vi "FlatToRichcif_manager_ClockUpdate.vi"(5 "OutputClusterType":T1, 11 "InputCluster":T3) -> (3 "OutputCluster":T1)   [LabVIEW 2021, in "CIF_Launcher_client.lvlib"]
uses:
  CIF_Launcher_client.lvlib
  cif_manager_ClockUpdate_Flat.ctl
  cif_manager_TimePair_Flat.ctl
  cif_manager_ClockUpdate.ctl
  cif_manager_TimePair.ctl
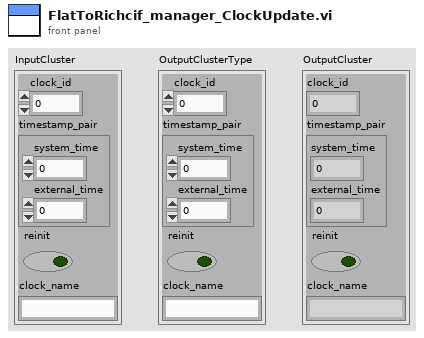
[diagram p1: front panel]
types:
  T1 = typedef "CIF_Launcher_client.lvlib/cif_manager_ClockUpdate.ctl" = cluster{"clock_id":u32, "timestamp_pair":T2, "reinit":bool, "clock_name":string}
  T2 = typedef "CIF_Launcher_client.lvlib/cif_manager_TimePair.ctl" = cluster{"system_time":i64, "external_time":i64}
  T3 = typedef "CIF_Launcher_client.lvlib/cif_manager_ClockUpdate_Flat.ctl" = cluster{"clock_id":u32, "timestamp_pair":T4, "reinit":bool, "clock_name":string}
  T4 = typedef "CIF_Launcher_client.lvlib/cif_manager_TimePair_Flat.ctl" = cluster{"system_time":i64, "external_time":i64}
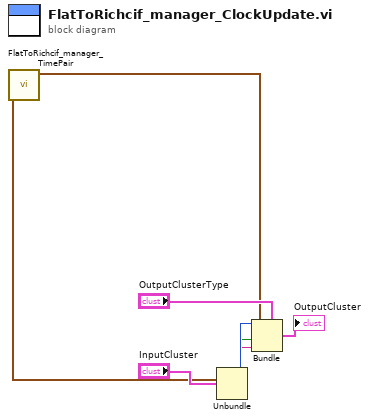
[diagram p0: block diagram]
diagram:
  n1 = Unbundle "Unbundle"("InputCluster") -> ("clock_id"=w5:u32, "timestamp_pair"=w4:T4, "reinit"=w2:bool, "clock_name"=w1:string)
  n2 = call "FlatToRichcif_manager_TimePair.vi"("InputCluster"=w4) -> ("OutputCluster"=w3:T2)  [unwired: 10 in]
  n3 = Bundle "Bundle"(cluster="OutputClusterType", "clock_id"=w5, "timestamp_pair"=w3, "reinit"=w2, "clock_name"=w1) -> (→"OutputCluster":T1)
